vi "Model Create.vi"(8 "error in (no error)":errorcluster) -> (0 "error out":errorcluster)   [LabVIEW 2015]
uses:
  Control Button/Exit.ctl
  Control Button/Save.ctl
  Control Button/Delete.ctl
  <vilib>/addons/database/Connection.llb/DB Tools Open Connec (String).vi
  Galobal variable_TI.vi
  <vilib>/addons/database/_DB Variant To Data/Database Variant To Data.xnode
  <vilib>/addons/database/NI_Database_API.lvlib
panel:
  out "new path":path
  out "Program seq. Name":string[](array[string])
  out "error out":errorcluster
  in  "Program Name":string
  in  "Edit Name":string
  in  "Program List":i32(listbox)
  in  "Delete":T1
  in  "Save":T2
  in  "Exit":T3
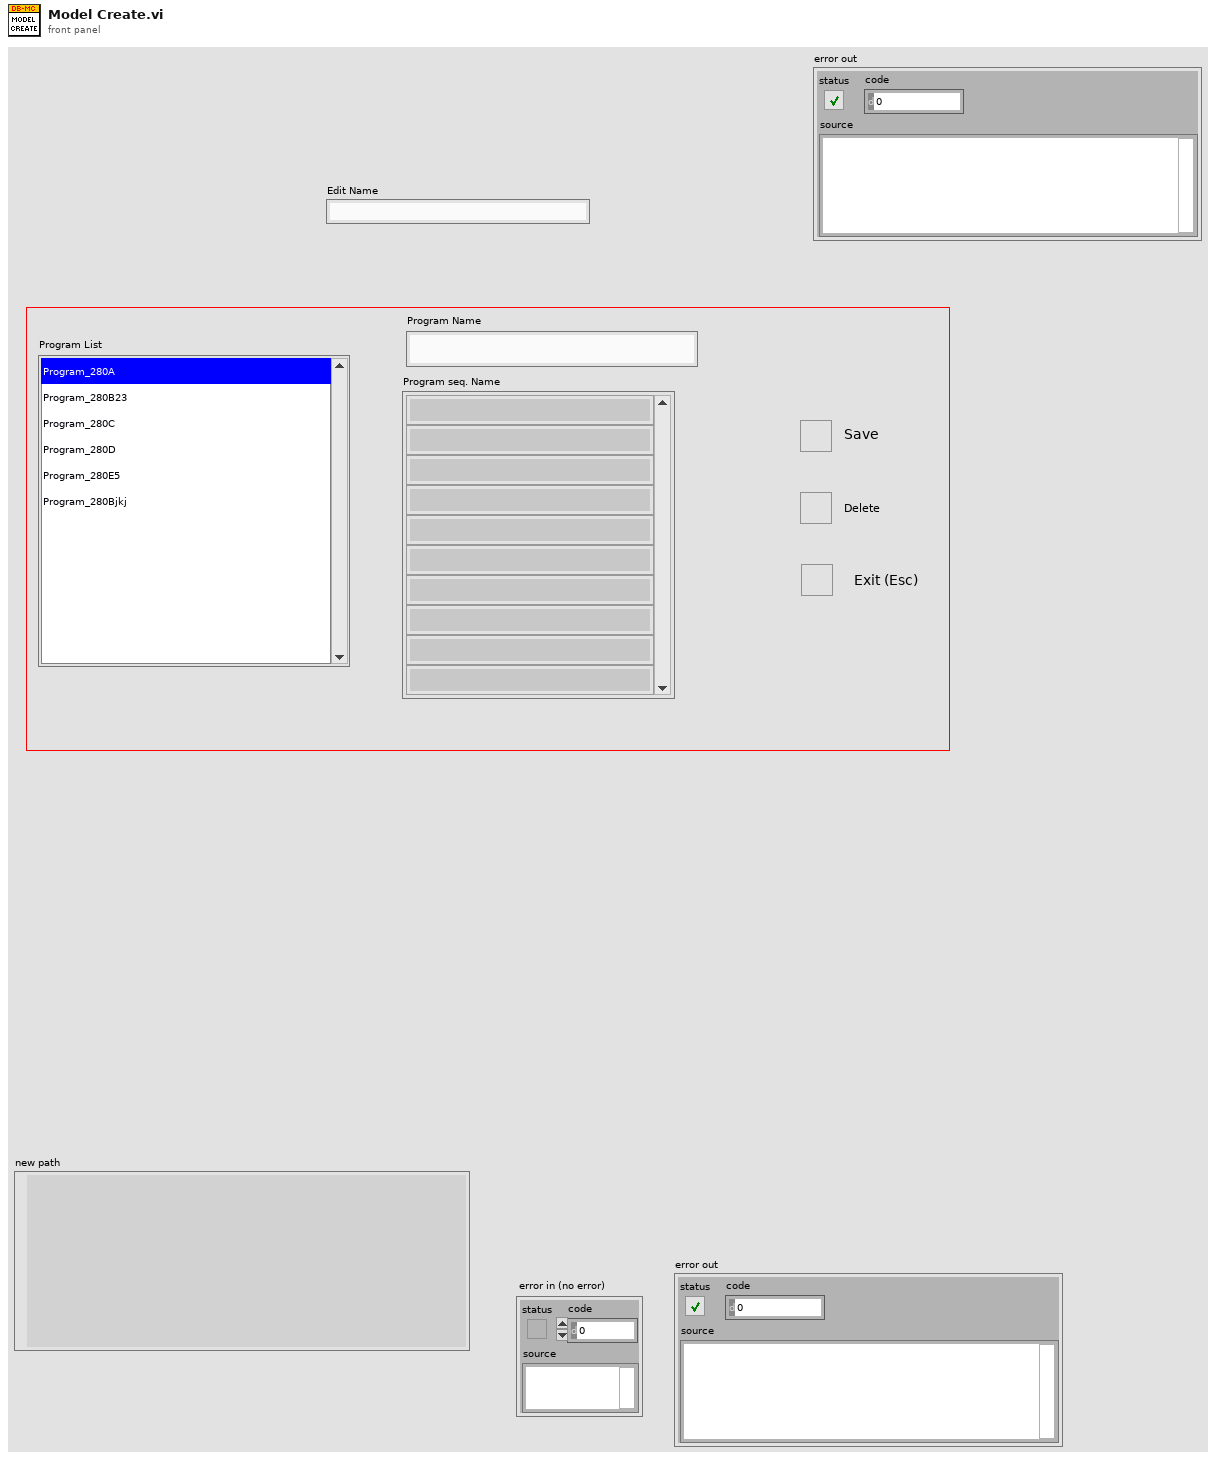
[diagram p1: front panel]
types:
  T1 = typedef "Delete.ctl" = bool
  T2 = typedef "Save.ctl" = bool
  T3 = typedef "Exit.ctl" = bool
  T4 = typedef "NI_Database_API.lvlib/Conn ObjectReference.ctl" = refnum<k1>
  T5 = enum16{"Left Button", "Center Button", "Right Button", "Window Close"}
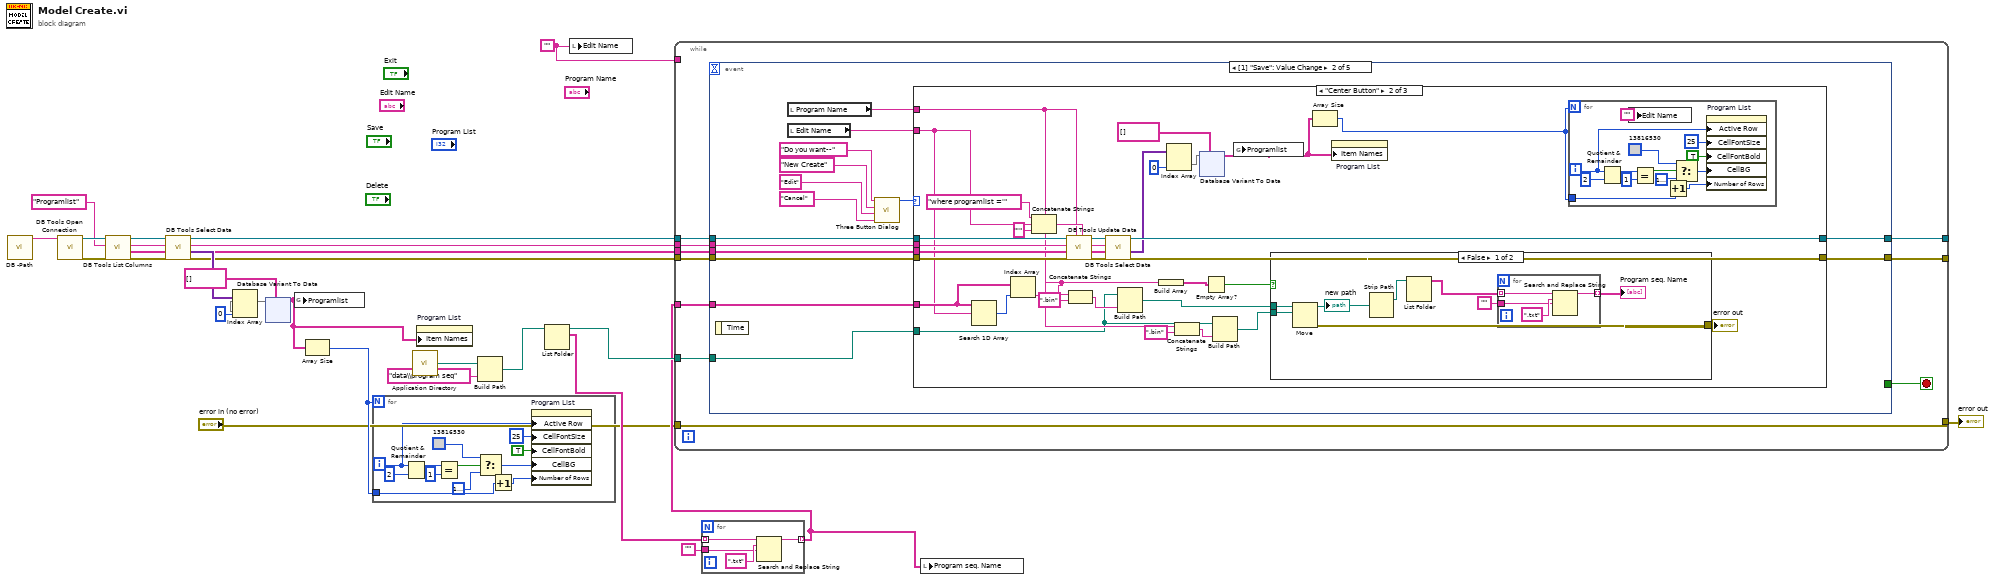
[diagram p0: block diagram]
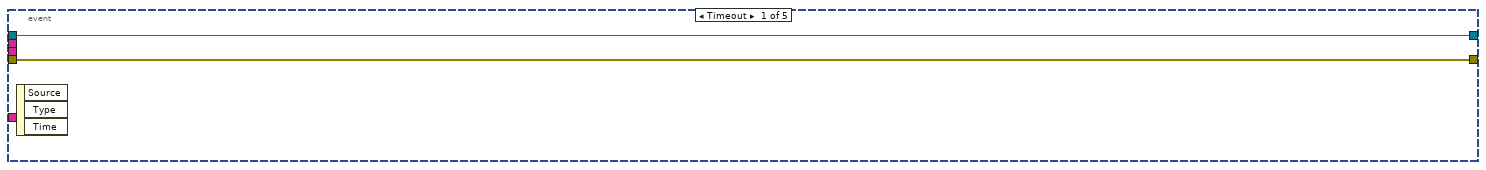
[diagram p2: hidden frame]
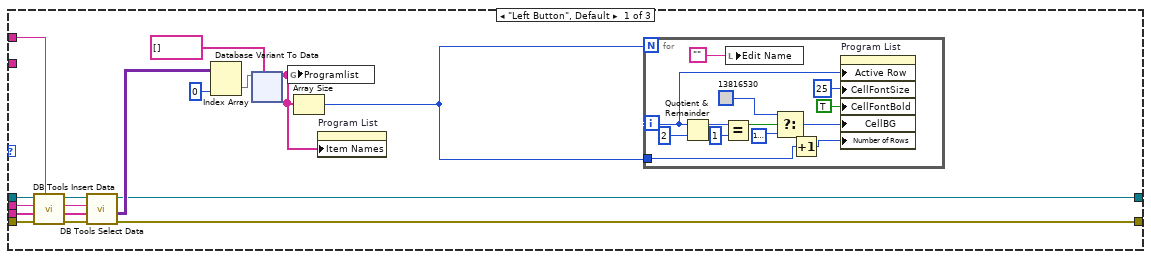
[diagram p3: hidden frame]
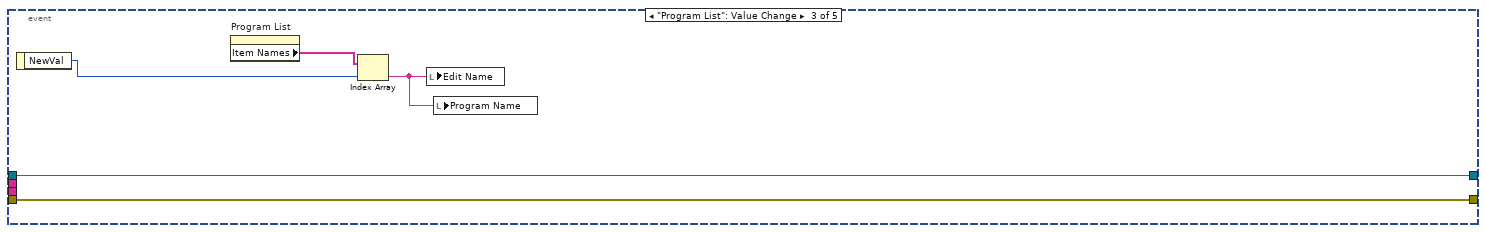
[diagram p6: hidden frame]
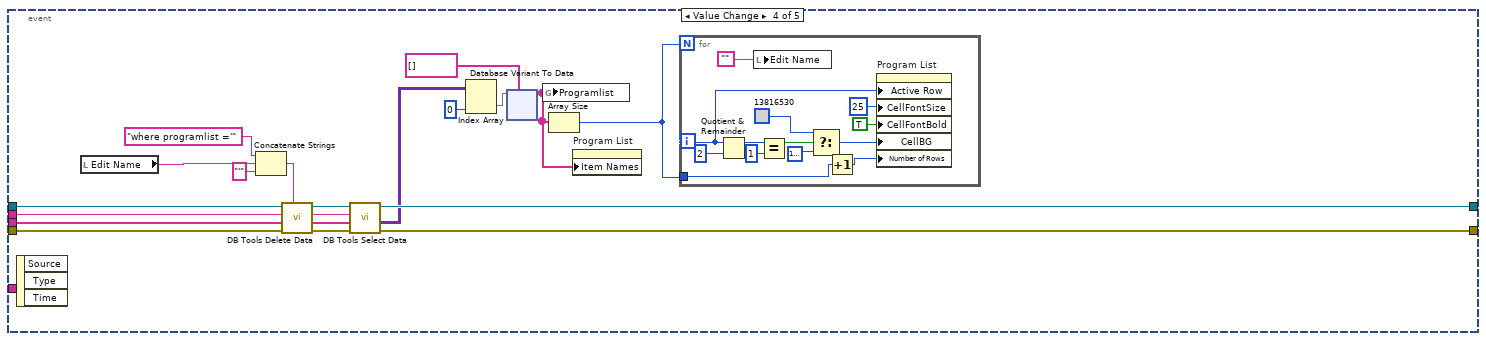
[diagram p7: hidden frame]
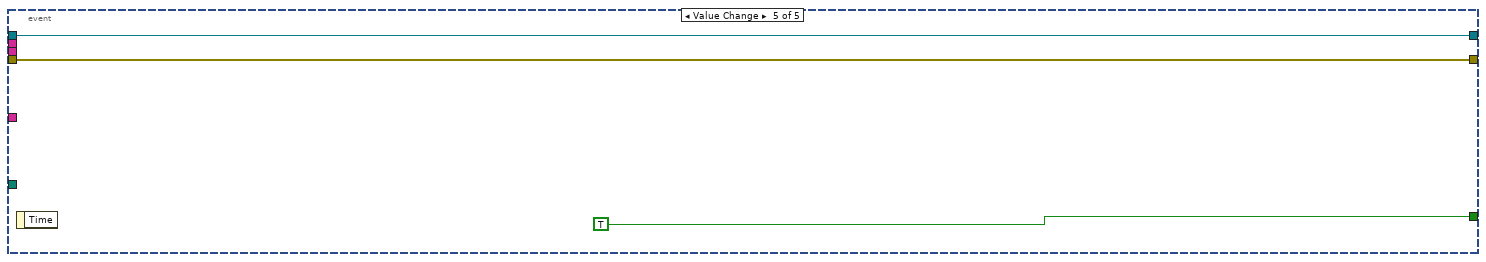
[diagram p8: hidden frame]
diagram:
  w8 = ""
  w11 = "Programlist" ("table")
  n1 = call "DB -Path.vi"() -> ("String"=w23:string)  [unwired: 11 in]
  n2 = call-poly <vilib>:"DB Tools Open Connection.vi"("connection information"=w23) -> ("error out"=w18:errorcluster, "connection reference"=w19:T4)  [unwired: 7 in]
  n3 = call <vilib>:"DB Tools List Columns.vi"("error in (no error)"=w18, "table"=w11, "connection reference"=w19) -> ("error out"=w16:errorcluster, "columns"=w12:string[], "connection reference out"=w17:T4)  [unwired: 1 in, 1 out]
  n4 = call <vilib>:"DB Tools Select Data.vi"("error in (no error)"=w16, "columns"=w12, "table"=w11, "connection reference"=w17) -> ("error out"=w13:errorcluster, "data"=w15:variant[][], "connection reference out"=w14:T4)  [unwired: 2 in]
  n5 = Index Array(array=w15, index (col)=0 ("disabled index (col)")) -> (element=w20:variant[])  [unwired: 1 in]
  n6 = xnode "Database Variant To Data"("database variant"=w20, "type"=string[] []) -> ("data"=w9:string[])  [unwired: 1 in, 1 out]
  n7 = global write "Galobal variable_TI.vi" "Programlist"(w9) -> ()
  n8 = Array Size(array=w9) -> (size(s)=w10:i32)
  n9 = for {
    N: w10 -> [_]
    tunnel: w10 -> [w27]
    i -> [w28]
    n10 = Quotient & Remainder(x=w28, y=2) -> (x-y*floor(x/y)=w36:i32)  [unwired: 1 out]
    n11 = Equal?(x=w36, y=1) -> (x = y?=w34:bool)
    n12 = Select(t=u32 13816530 ("Color Box"), s=w34, f=u32 16777225 ("Color Box")) -> (s? t:f=w31:u32)
    n13 = Increment(x=w27) -> (x+1=w26:i32)
    n14 = property on="Program List" class="LstBox (strict)"("Active Row"=w28, "CellFontSize"=u32 25 ("Active Row:Cell Font:Size"), "CellFontBold"=TRUE ("Active Row:Cell Font:Bold"), "CellBG"=w31, "Number of Rows"=w26) -> ()  [unwired: 2 in, 2 out]
  }
  n15 = call <vilib>:"Application Directory.vi"() -> ("Application Directory"=w25:path)
  n16 = property on="Program List" class="LstBox (strict)"("Item Names"=w9) -> ()  [unwired: 2 in, 2 out]
  n17 = Build Path(base path=w25, name or relative path="data\\program seq") -> (appended path=w7:path)
  n18 = List Folder(path=w7) -> (path out=w6:path, filenames=w5:string[])  [unwired: 3 in, 2 out]
  n19 = local write "Edit Name"(w8) -> ()
  n20 = for {
    tunnel: w5 -> [w41] mode=indexing
    tunnel: "" -> [w39]
    tunnel: [w38] -> w3 mode=indexing
    n21 = Search and Replace String(input string=w41, search string=".txt" ("replace string (\"\")"), replace string=w39) -> (result string=w38:string)  [unwired: 5 in, 3 out]
  }
  n22 = while {
    tunnel: w6 -> [w50]
    tunnel: w14 -> [w49]
    tunnel: w13 -> [w48]
    tunnel: w12 -> [w47]
    tunnel: w11 -> [w46]
    tunnel: [w45] -> _
    tunnel: [w44] -> _
    tunnel: w8 -> [_]
    tunnel: w3 -> [w43]
    tunnel: [w42] -> w2
    tunnel: "error in (no error)" -> [w42]
    stop <- w51 stop-if-true
    n23 = event shown="[1] \"Save\": Value Change" {
      selector: _ -> [_ _ _ _ _]
      dyn-events: _ -> [_ _ _ _ _]
      timeout: _ -> [_ _ _ _ _]
      tunnel: [_ _ _ _ TRUE] -> w51
      tunnel: w50 -> [_ w55 _ _ _]
      tunnel: w49 -> [w53 w63 w236 w254 w307]
      tunnel: w48 -> [w52 w62 w235 w253 w306]
      tunnel: w47 -> [_ w60 _ w249 _]
      tunnel: w46 -> [_ w61 _ w250 _]
      tunnel: [w53 w59 w236 w248 w307] -> w45
      tunnel: [w52 w58 w235 w247 w306] -> w44
      tunnel: w43 -> [_ w56 _ _ _]
      event Timeout {
        n24 = event-data() -> ()  [unwired: 1 in, 3 out]
      }
      event Value Change {
        n25 = event-data() -> ()  [unwired: 1 in, 1 out]
        n26 = local read "Program Name"() -> (w54:string)
        n27 = local read "Edit Name"() -> (w57:string)
        n28 = call <vilib>:"Three Button Dialog.vi"("Right Button Text (\"Cancel\")"="Cancel" ("Right Button Text (\"Cancel\")"), "Center Button Text (\"No\")"="Edit" ("Center Button Text (\"No\")"), "Left Button Text (\"Yes\")"="New Create" ("Left Button Text (\"Yes\")"), "message"="Do you want--" ("Left Button Text (\"Yes\")")) -> ("Which Button?"=w68:T5)  [unwired: 7 in]
        n29 = case shown="\"Center Button\"" w68 {
          tunnel: w63 -> [w83 w166 w231]
          tunnel: w62 -> [w82 w165 w230]
          tunnel: w61 -> [w79 w159 _]
          tunnel: w60 -> [w78 w158 _]
          tunnel: [w72 w157 w231] -> w59
          tunnel: [w71 w156 w230] -> w58
          tunnel: w57 -> [_ w145 _]
          tunnel: w56 -> [_ w149 _]
          tunnel: w55 -> [_ w138 _]
          tunnel: w54 -> [w69 w139 _]
          frame "Left Button", Default {
            n30 = call <vilib>:"DB Tools Insert Data.vi"("data"=w69, "error in (no error)"=w82, "columns"=w78, "table"=w79, "connection reference"=w83) -> ("error out"=w80:errorcluster, "connection reference out"=w81:T4)  [unwired: 5 in]
            n31 = call <vilib>:"DB Tools Select Data.vi"("error in (no error)"=w80, "columns"=w78, "table"=w79, "connection reference"=w81) -> ("error out"=w71:errorcluster, "data"=w74:variant[][], "connection reference out"=w72:T4)  [unwired: 2 in]
            n32 = Index Array(array=w74, index (col)=0 ("disabled index (col)")) -> (element=w77:variant[])  [unwired: 1 in]
            n33 = xnode "Database Variant To Data"("database variant"=w77, "type"=string[] []) -> ("data"=w70:string[])  [unwired: 1 in, 1 out]
            n34 = global write "Galobal variable_TI.vi" "Programlist"(w70) -> ()
            n35 = Array Size(array=w70) -> (size(s)=w73:i32)
            n36 = property on="Program List" class="LstBox (strict)"("Item Names"=w70) -> ()  [unwired: 2 in, 2 out]
            n37 = for {
              N: w73 -> [_]
              tunnel: w73 -> [w86]
              i -> [w87]
              n38 = Quotient & Remainder(x=w87, y=2) -> (x-y*floor(x/y)=w95:i32)  [unwired: 1 out]
              n39 = Equal?(x=w95, y=1) -> (x = y?=w93:bool)
              n40 = local write "Edit Name"("") -> ()
              n41 = Select(t=u32 13816530 ("Color Box"), s=w93, f=u32 16777225 ("Color Box")) -> (s? t:f=w90:u32)
              n42 = Increment(x=w86) -> (x+1=w85:i32)
              n43 = property on="Program List" class="LstBox (strict)"("Active Row"=w87, "CellFontSize"=u32 25 ("Active Row:Cell Font:Size"), "CellFontBold"=TRUE ("Active Row:Cell Font:Bold"), "CellBG"=w90, "Number of Rows"=w85) -> ()  [unwired: 2 in, 2 out]
            }
          }
          frame "Center Button" {
            n44 = Search 1D Array(1D array=w149, element=w145) -> (index of element=w148:i32)  [unwired: 1 in]
            n45 = Index Array(array=w149, index=w148) -> (element=w144:string)
            n46 = Concatenate Strings("where programlist ='" ("condition"), w145, "'" ("string")) -> (w164:string)
            n47 = call <vilib>:"DB Tools Update Data.vi"("condition"=w164, "data"=w139, "error in (no error)"=w165, "columns"=w158, "table"=w159, "connection reference"=w166) -> ("error out"=w160:errorcluster, "connection reference out"=w161:T4)  [unwired: 4 in]
            n48 = Concatenate Strings(w144, ".bin" ("string")) -> (w142:string)
            n49 = call <vilib>:"DB Tools Select Data.vi"("error in (no error)"=w160, "columns"=w158, "table"=w159, "connection reference"=w161) -> ("error out"=w156:errorcluster, "data"=w150:variant[][], "connection reference out"=w157:T4)  [unwired: 2 in]
            n50 = Build Path(base path=w138, name or relative path=w142) -> (appended path=w141:path)
            n51 = Build Array(w144) -> (w147:string[])
            n52 = Index Array(array=w150, index (col)=0 ("disabled index (col)")) -> (element=w155:variant[])  [unwired: 1 in]
            n53 = Concatenate Strings(w139, ".bin" ("string")) -> (w137:string)
            n54 = xnode "Database Variant To Data"("database variant"=w155, "type"=string[] []) -> ("data"=w151:string[])  [unwired: 1 in, 1 out]
            n55 = Empty Array?(array=w147) -> (empty?=w146:bool)
            n56 = Build Path(base path=w138, name or relative path=w137) -> (appended path=w136:path)
            n57 = global write "Galobal variable_TI.vi" "Programlist"(w151) -> ()
            n58 = case shown="False" w146 {
              tunnel: w141 -> [w174 _]
              tunnel: w136 -> [w173 _]
              tunnel: [w172 _] -> w135
              frame False {
                n59 = Move(source path=w174, 10:w173) -> (error out=w172:errorcluster, 3:w171:path)  [unwired: 3 in, 1 out]
                "new path" <- w171
                n60 = Strip Path(path=w171) -> (stripped path=w170:path)  [unwired: 1 out]
                n61 = List Folder(path=w170) -> (filenames=w168:string[])  [unwired: 3 in, 3 out]
                n62 = for {
                  tunnel: w168 -> [w178] mode=indexing
                  tunnel: "" -> [w176]
                  tunnel: [w175] -> w167 mode=indexing
                  n63 = Search and Replace String(input string=w178, search string=".txt" ("replace string (\"\")"), replace string=w176) -> (result string=w175:string)  [unwired: 5 in, 3 out]
                }
                "Program seq. Name" <- w167
              }
              frame True {
              }
            }
            "error out" <- w135
            n64 = Array Size(array=w151) -> (size(s)=w152:i32)
            n65 = property on="Program List" class="LstBox (strict)"("Item Names"=w151) -> ()  [unwired: 2 in, 2 out]
            n66 = for {
              N: w152 -> [_]
              tunnel: w152 -> [w181]
              i -> [w182]
              n67 = Quotient & Remainder(x=w182, y=2) -> (x-y*floor(x/y)=w190:i32)  [unwired: 1 out]
              n68 = local write "Edit Name"("") -> ()
              n69 = Equal?(x=w190, y=1) -> (x = y?=w188:bool)
              n70 = Increment(x=w181) -> (x+1=w180:i32)
              n71 = Select(t=u32 13816530 ("Color Box"), s=w188, f=u32 16777225 ("Color Box")) -> (s? t:f=w185:u32)
              n72 = property on="Program List" class="LstBox (strict)"("Active Row"=w182, "CellFontSize"=u32 25 ("Active Row:Cell Font:Size"), "CellFontBold"=TRUE ("Active Row:Cell Font:Bold"), "CellBG"=w185, "Number of Rows"=w180) -> ()  [unwired: 2 in, 2 out]
            }
          }
          frame "Right Button" {
          }
        }
      }
      event "Program List": Value Change {
        n73 = event-data() -> ("NewVal"=w233:i32)  [unwired: 1 in]
        n74 = property on="Program List" class="LstBox (strict)"() -> ("Item Names"=w234:string[])  [unwired: 2 in, 2 out]
        n75 = Index Array(array=w234, index=w233) -> (element=w232:string)
        n76 = local write "Edit Name"(w232) -> ()
        n77 = local write "Program Name"(w232) -> ()
      }
      event Value Change {
        n78 = event-data() -> ()  [unwired: 1 in, 3 out]
        n79 = local read "Edit Name"() -> (w237:string)
        n80 = Concatenate Strings("where programlist ='" ("condition"), w237, "'" ("string")) -> (w238:string)
        n81 = call <vilib>:"DB Tools Delete Data.vi"("condition"=w238, "error in (no error)"=w253, "table"=w250, "connection reference"=w254) -> ("error out"=w251:errorcluster, "connection reference out"=w252:T4)  [unwired: 6 in]
        n82 = call <vilib>:"DB Tools Select Data.vi"("error in (no error)"=w251, "columns"=w249, "table"=w250, "connection reference"=w252) -> ("error out"=w247:errorcluster, "data"=w241:variant[][], "connection reference out"=w248:T4)  [unwired: 2 in]
        n83 = Index Array(array=w241, index (col)=0 ("disabled index (col)")) -> (element=w246:variant[])  [unwired: 1 in]
        n84 = xnode "Database Variant To Data"("database variant"=w246, "type"=string[] []) -> ("data"=w242:string[])  [unwired: 1 in, 1 out]
        n85 = global write "Galobal variable_TI.vi" "Programlist"(w242) -> ()
        n86 = Array Size(array=w242) -> (size(s)=w243:i32)
        n87 = property on="Program List" class="LstBox (strict)"("Item Names"=w242) -> ()  [unwired: 2 in, 2 out]
        n88 = for {
          N: w243 -> [_]
          tunnel: w243 -> [w257]
          i -> [w258]
          n89 = Quotient & Remainder(x=w258, y=2) -> (x-y*floor(x/y)=w266:i32)  [unwired: 1 out]
          n90 = local write "Edit Name"("") -> ()
          n91 = Equal?(x=w266, y=1) -> (x = y?=w264:bool)
          n92 = Select(t=u32 13816530 ("Color Box"), s=w264, f=u32 16777225 ("Color Box")) -> (s? t:f=w261:u32)
          n93 = Increment(x=w257) -> (x+1=w256:i32)
          n94 = property on="Program List" class="LstBox (strict)"("Active Row"=w258, "CellFontSize"=u32 25 ("Active Row:Cell Font:Size"), "CellFontBold"=TRUE ("Active Row:Cell Font:Bold"), "CellBG"=w261, "Number of Rows"=w256) -> ()  [unwired: 2 in, 2 out]
        }
      }
      event Value Change {
        n95 = event-data() -> ()  [unwired: 1 in, 1 out]
      }
    }
  }
  "error out" <- w2
  n96 = local write "Program seq. Name"(w3) -> ()
